vi "Write Module Page Property.vi"(8 "error in (no error)":errorcluster, 10 "RSI Module":refnum<class "RSI Module.lvclass">, 11 "Node Ptr In":T1 format="%.0x") -> (0 "error out":errorcluster, 2 "RSI Module out":refnum<class "RSI Module.lvclass">, 3 "Node Ptr Out":T1 format="%.0x")   [LabVIEW 2017, in "Modules.lvlib" / "RSI Module.lvclass"]
uses:
  RSI Module.lvclass
  <vilib>/NI Veristand/Custom Device API/Custom Device Item Ref.ctl
  Debug.vi
  Class Property Strings.vi
  <vilib>/NI Veristand/Custom Device API/Set Item Property (String).vi
  <vilib>/NI Veristand/Custom Device API/Custom Device API.lvlib
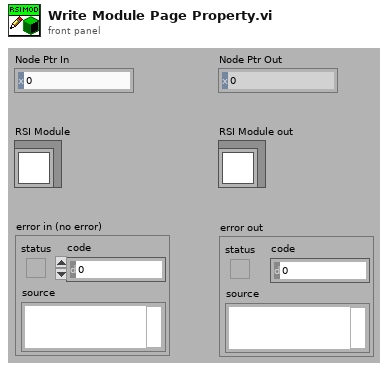
[diagram p1: front panel]
types:
  T1 = typedef "Custom Device API.lvlib/Custom Device Item Ref.ctl" = u64
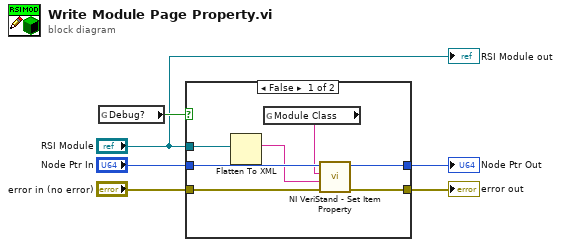
[diagram p0: block diagram]
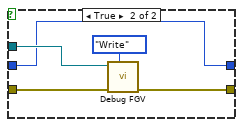
[diagram p2: hidden frame]
diagram:
  n1 = global read "Debug.vi" "Debug?"() -> (w2:bool)
  n2 = case shown="False" w2 {
    tunnel: "Node Ptr In" -> [w13 w14]
    tunnel: [w12 w14] -> w5
    tunnel: [w11 w15] -> w4
    tunnel: "RSI Module" -> [w9 w16]
    tunnel: "error in (no error)" -> [w7 w17]
    frame False {
      n3 = Flatten To XML(anything=w9) -> (xml string=w8:string)
      n4 = global read "Class Property Strings.vi" "Module Class"() -> (w10:string)
      n5 = call-poly <vilib>:"NI VeriStand - Set Item Property.vi"("error in (no error)"=w7, "Value"=w8, "Property Name"=w10, "Item Ref in"=w13) -> ("error out"=w11:errorcluster, "Item Ref out"=w12:T1)  [unwired: 5 in, 1 out]
    }
    frame True {
      n6 = call "Debug FGV.vi"("Action"=enum16{"Read", "Write"}."Write", "error in (no error)"=w17, "RSI Module in"=w16) -> ("error out"=w15:errorcluster)  [unwired: 7 in, 1 out]
    }
  }
  "Node Ptr Out" <- w5
  "error out" <- w4
  "RSI Module out" <- "RSI Module"
